vi "Get Front End Status.vi"(11 "piFlag":i32) -> (2 "function return":u32, 3 "piFlag out":i32)   [LabVIEW 2018, in "AndorSDK.lvlib"]
doc: "EXPNETTYPE unsigned int WINAPI GetFrontEndStatus(int * piFlag);"
uses:
  AndorSDK.lvlib
  ATMCD32D.dll
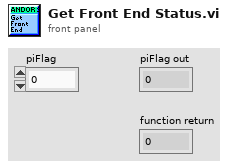
[diagram p1: front panel]
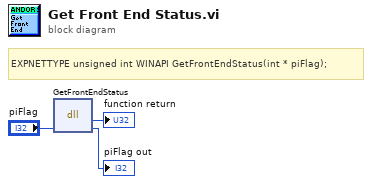
[diagram p0: block diagram]
diagram:
  # "EXPNETTYPE unsigned int WINAPI GetFrontEndStatus(int * piFlag);"
  n1 = dll-call lib="PTH2babs E\nPersönliches02 - Arbeit03-HiwijobsLabviewCodelibANDOR\tAndor SDK\nATMCD32D.*" fn="GetFrontEndStatus"("piFlag"="piFlag") -> (→"function return":u32, "piFlag"=→"piFlag out":i32)  [unwired: 3 in, 2 out]
